vi "Read Attributes.vi"(11 "Time Info Msg":refnum<class "Time Info Msg.lvclass">) -> (2 "Payload":cluster{"Elapsed?":bool, "Elapsed Time":dbl})   [LabVIEW 2019, in "Timer.lvlib" / "Time Info Msg.lvclass"]
uses:
  Time Info Msg.lvclass
  Time Info Msg.lvclass/Time Info Msg.ctl
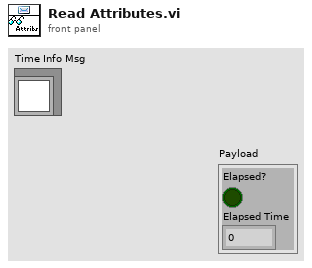
[diagram p1: front panel]
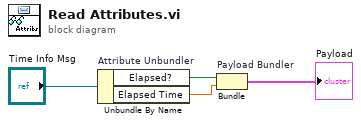
[diagram p0: block diagram]
diagram:
  n1 = Unbundle By Name "Attribute Unbundler"("Time Info Msg") -> ("Elapsed?"=w2:bool, "Elapsed Time"=w1:dbl)
  n2 = Bundle "Payload Bundler"("Elapsed?"=w2, "Elapsed Time"=w1) -> (→"Payload":cluster{"Elapsed?":bool, "Elapsed Time":dbl})  [unwired: 1 in]
